vi "dialog_box for calibration.vi"(8 "error in (no error)":errorcluster caption="错误输入（无错误）") -> (0 "error out":errorcluster caption="错误输出", 2 "parameter for calibration out":T1={"分子长度（bp）"=0, "磁球大小（直径）"=0.0, "校准起点"=0.0, "校准步长"=0.0, "每步采样数（frame）"=0, "首尾去除帧数(frame)"=0, "校准步数"=0, "底面位置"=0.0, "R-step"=1.0, "R-min"=0.0, "R-max"=0.0, "num"=2, "x_center"=0.0, "y_center"=0.0, "磁铁位置"=0.0}, 3 "Cancelled?":bool caption="取消？")   [LabVIEW 2013]
doc: "该模板用于创建能够进行事件处理的对话框。"
uses:
  parameter set for calibration.ctl
panel:
  in  "parameter for calibration":T1={"分子长度（bp）"=0, "磁球大小（直径）"=0.0, "校准起点"=0.0, "校准步长"=0.0, "每步采样数（frame）"=0, "首尾去除帧数(frame)"=0, "校准步数"=0, "底面位置"=0.0, "R-step"=1.0, "R-min"=0.0, "R-max"=0.0, "num"=2, "x_center"=0.0, "y_center"=0.0, "磁铁位置"=0.0}
  in  "底面位置":dbl
  in  "校准步数":dbl
  in  "首尾去除帧数(frame)":i32
  in  "每步采样数（frame）":i32
  in  "校准步长":dbl
  in  "校准起点":dbl
  in  "磁球大小（直径）":dbl[unit]
  in  "分子长度（bp）":i32
  in  "Cancel":bool caption="取消"
  in  "OK":bool caption="确定"
  # "校准参数设置"
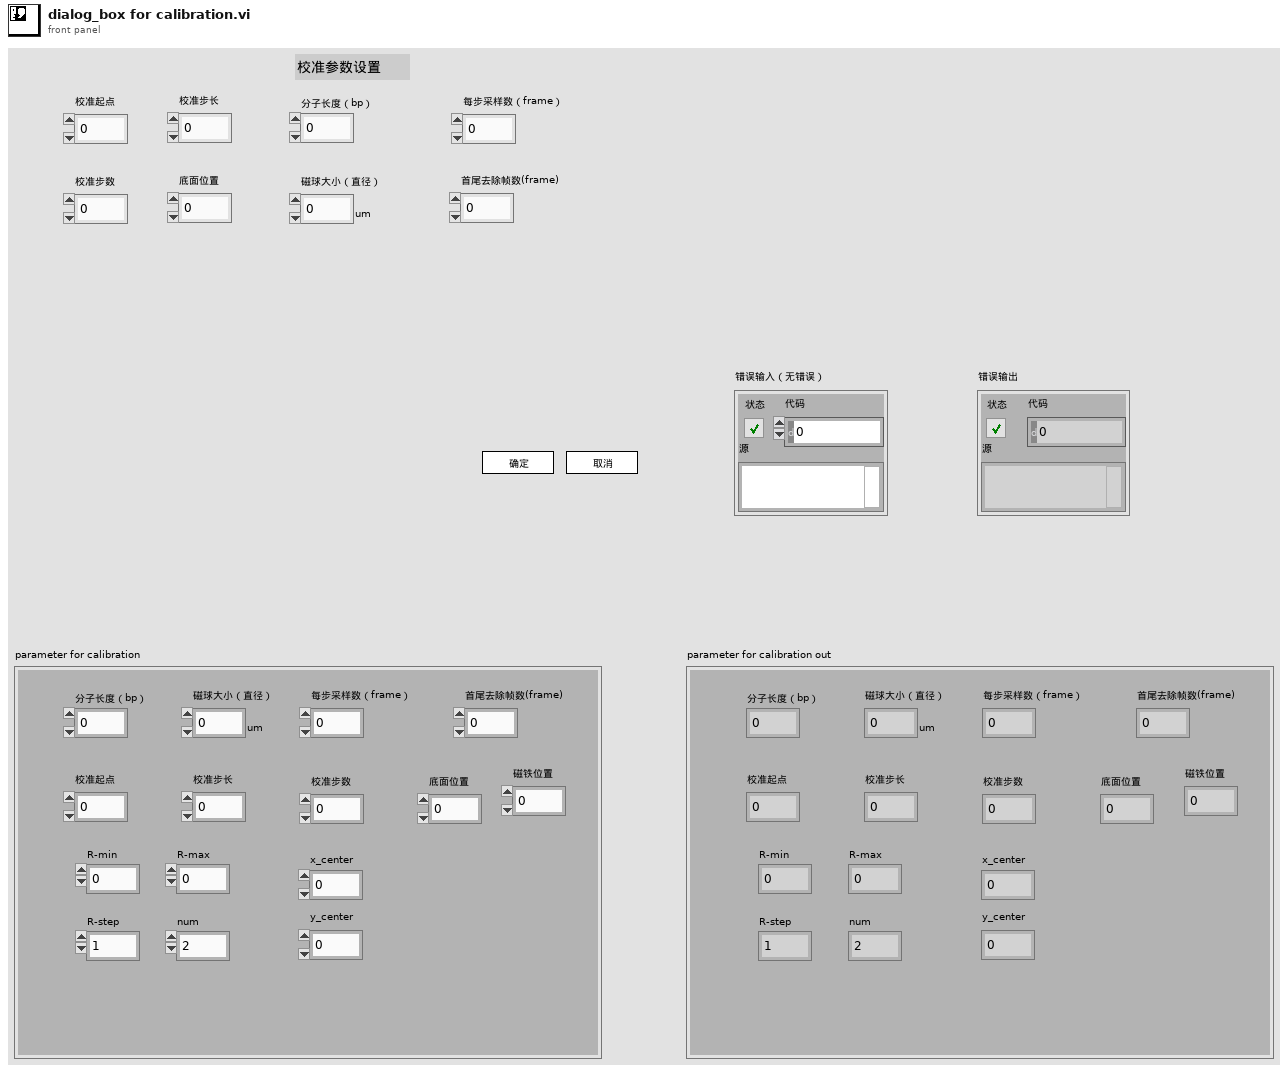
[diagram p1: front panel]
types:
  T1 = typedef "parameter set for calibration.ctl" = cluster{"分子长度（bp）":i32, "磁球大小（直径）":dbl[unit], "校准起点":dbl, "校准步长":dbl, "每步采样数（frame）":i32, "首尾去除帧数(frame)":i32, "校准步数":i32, "底面位置":dbl, "R-step":sgl, "R-min":sgl, "R-max":sgl, "num":i32, "x_center":dbl, "y_center":dbl, "磁铁位置":dbl}
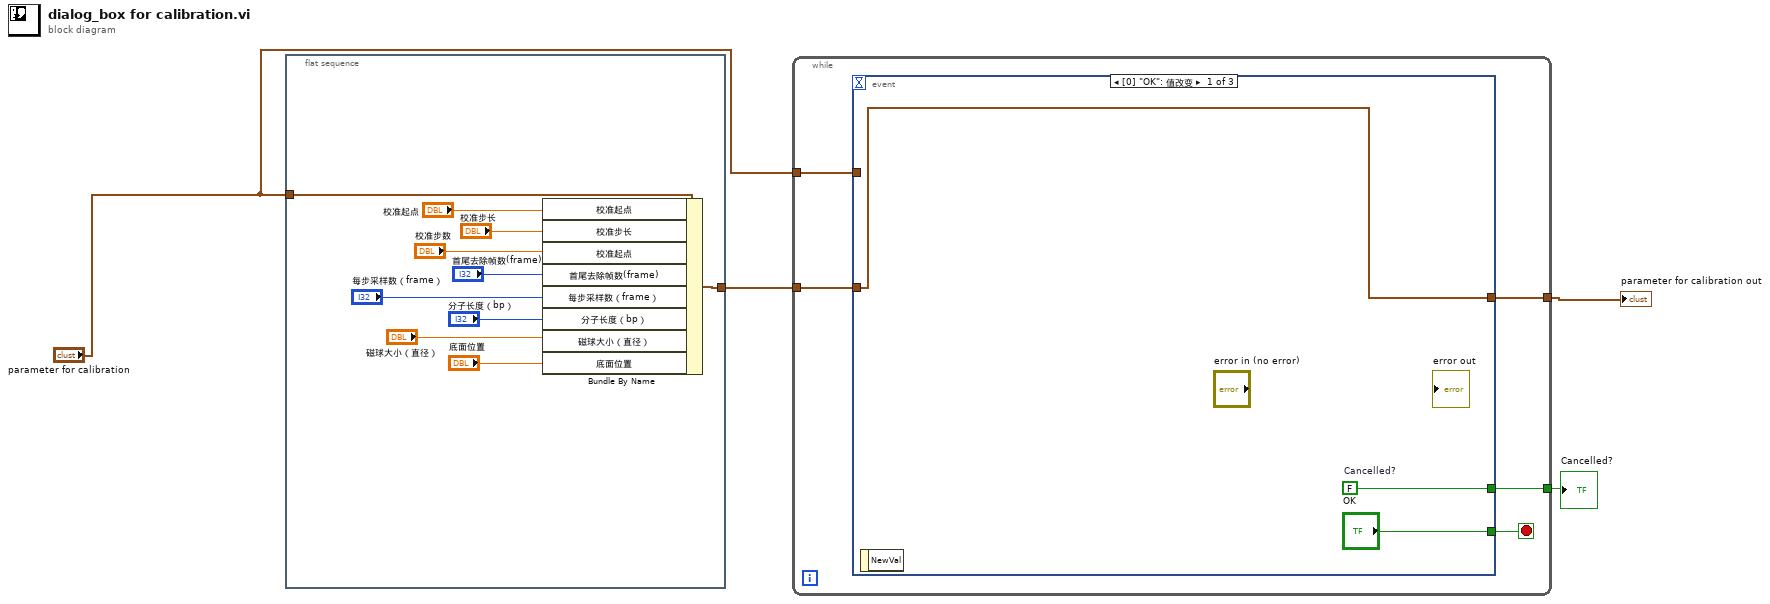
[diagram p0: block diagram]
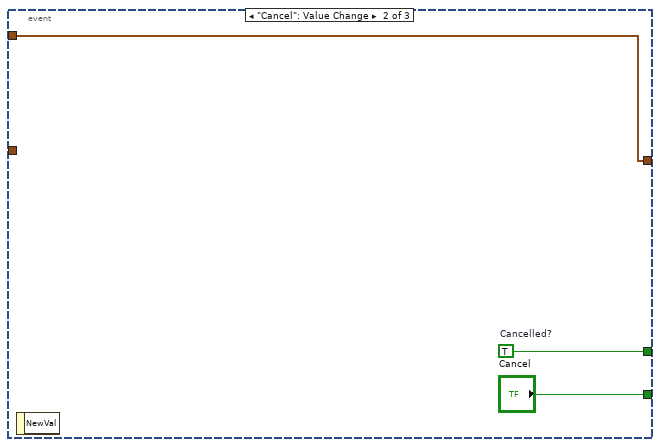
[diagram p2: hidden frame]
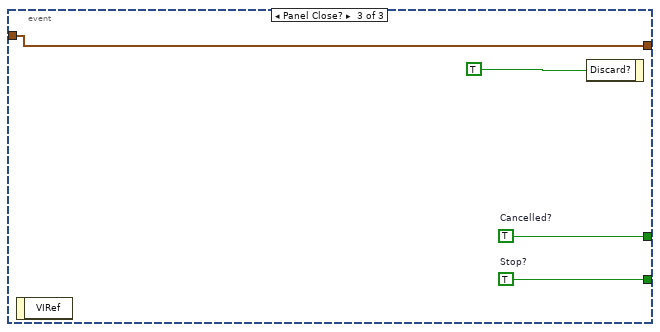
[diagram p3: hidden frame]
diagram:
  n1 = flat-sequence {
    tunnel: "parameter for calibration" -> [w14]
    tunnel: [w13] -> w3
    frame #0 {
      n2 = Bundle By Name(cluster=w14, "校准起点"="校准起点", "校准步长"="校准步长", "校准起点"="校准步数", "首尾去除帧数(frame)"="首尾去除帧数(frame)", "每步采样数（frame）"="每步采样数（frame）", "分子长度（bp）"="分子长度（bp）", "磁球大小（直径）"="磁球大小（直径）", "底面位置"="底面位置") -> (w13:T1)
    }
  }
  n3 = while {
    tunnel: [w18] -> w4
    tunnel: w3 -> [w17]
    tunnel: [w16] -> w2
    tunnel: "parameter for calibration" -> [w15]
    stop <- w19 stop-if-true
    n4 = event shown="[0] \"OK\": 值改变" {
      selector: _ -> [_ _ _]
      dyn-events: _ -> [_ _ _]
      timeout: _ -> [_ _ _]
      tunnel: ["OK" "Cancel" w28] -> w19
      tunnel: [w22 w25 w27] -> w18
      tunnel: w17 -> [w20 _ w26]
      tunnel: [w20 w23 w26] -> w16
      tunnel: w15 -> [_ w23 _]
      event "OK": Value Change {
        w22 = FALSE  # Cancelled?
        n5 = event-data() -> ()  [unwired: 1 in, 1 out]
      }
      event "Cancel": Value Change {
        w25 = TRUE  # Cancelled?
        n6 = event-data() -> ()  [unwired: 1 in, 1 out]
      }
      event Panel Close? {
        w27 = TRUE  # Cancelled?
        w28 = TRUE  # Stop?
        n7 = event-data() -> ()  [unwired: 1 in, 1 out]
        n8 = event-data("Discard?"=TRUE) -> ()  [unwired: 1 in, 1 out]
      }
    }
  }
  "Cancelled?" <- w4
  "parameter for calibration out" <- w2
